vi "File_Test.vi"() -> ()   [LabVIEW 2013]
uses:
  experimentData.ctl
  File_Module Control.ctl
panel:
  in  "All Data":T1={"elapsedTime"=10.0, "forwardPower"=20.0, "reversePower"=30.0, "temperature"=40.0} {"temperature" format="%#.1g"; "elapsedTime" format="%#.1g"; "reversePower" format="%#.1g"; "forwardPower" format="%#.1g"}
  out "Ciclo":i32
  out "error out":errorcluster
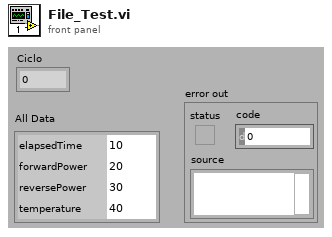
[diagram p1: front panel]
types:
  T1 = typedef "experimentData.ctl" = cluster{"elapsedTime":dbl, "forwardPower":dbl, "reversePower":dbl, "temperature":dbl}
  T2 = typedef "File_Module Control.ctl" = enum16{"Initialize", "Save Head", "Save Data", "Shutdown"}
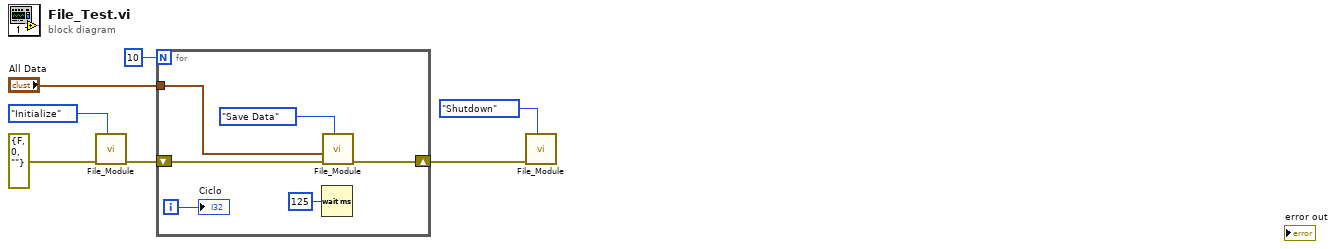
[diagram p0: block diagram]
diagram:
  n1 = call "File_Module.vi"("Command"=File_Module_Control."Initialize", "error in (no error)"=errorcluster {"status"=FALSE, "code"=0, "source"=""}) -> ("error out"=w6:errorcluster)  [unwired: 9 in]
  n2 = for {
    N: 10 -> [_]
    shift-right: [w8] -> w2
    shift-left: w6 -> [w11]
    tunnel: "All Data" -> [w9]
    i -> [w12]
    n3 = Wait (ms)(milliseconds to wait=u32 125) -> ()  [unwired: 1 out]
    n4 = call "File_Module.vi"("Command"=File_Module_Control."Save Data", "error in (no error)"=w11, "All Data"=w9) -> ("error out"=w8:errorcluster)  [unwired: 8 in]
    "Ciclo" <- w12
  }
  n5 = call "File_Module.vi"("Command"=File_Module_Control."Shutdown", "error in (no error)"=w2) -> ()  [unwired: 9 in, 1 out]
